vi "Laurel StandAlone TCP.vi"() -> ()   [LabVIEW 2016]
uses:
  Type Definitions/Laurel Serial Commands.ctl
  Type Definitions/Laurel Connection Type.ctl
panel:
  in  "stop":bool
  out "Single Item":dbl
  out "Gallons (Item 2)":dbl
  out "Flow Rate (Item 1)":dbl format="%.2f"
  in  "All Items Byte Count (Flow Rate)":i32=17
  in  "byte count (Individual)":i32=8
  in  "Laurel Serial Commands":T1
  out "read buffer":string
  out "Error Out 2":errorcluster
  in  "Error In 2":errorcluster
  in  "Hot Laurel Only":string="10.2.0.23"
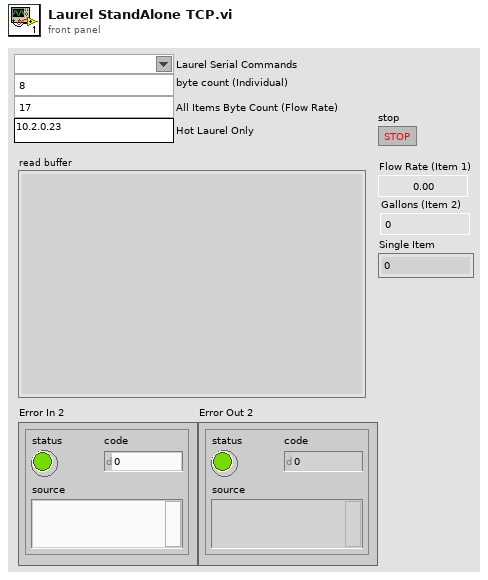
[diagram p1: front panel]
types:
  T1 = typedef "Laurel Serial Commands.ctl" = string
  T2 = typedef "Laurel Connection Type.ctl" = enum16{"Serial", "TCP"}
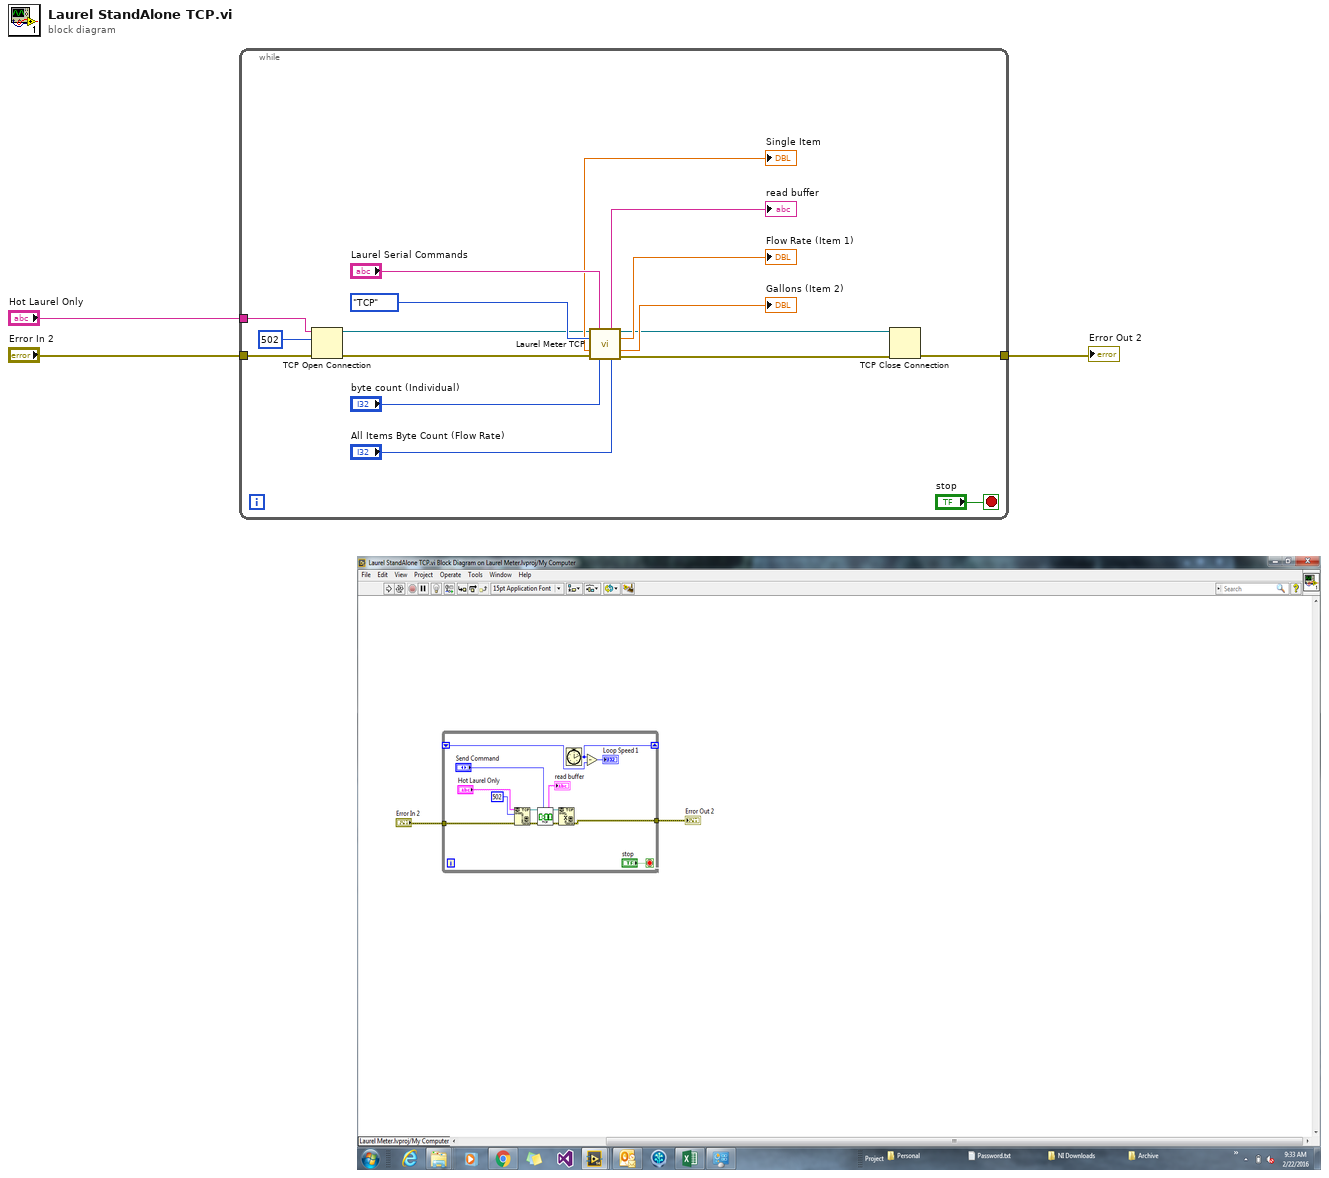
[diagram p0: block diagram]
diagram:
  n1 = while {
    tunnel: "Hot Laurel Only" -> [w9]
    tunnel: "Error In 2" -> [w8]
    tunnel: [w4] -> w1
    stop <- "stop" stop-if-true
    n2 = TCP Open Connection(address=w9, remote port or service name=u16 502, error in (no error)=w8) -> (connection ID=w7:refnum<k5>, error out=w10:errorcluster)  [unwired: 2 in]
    n3 = call "Laurel Meter TCP.vi"("TCP Network Connection in"=w7, "Laurel Serial Commands"="Laurel Serial Commands", "Connection Type"=Laurel_Connection_Type."TCP", "error in (no error)"=w10, "byte count (Individual)"="byte count (Individual)", "All Items Byte Count (Flow Rate)"="All Items Byte Count (Flow Rate)") -> ("read buffer"=→"read buffer":string, "TCP Network Connection out"=w5:refnum<k5>, "Flow Rate (Item 1)"=→"Flow Rate (Item 1)":dbl, "Single Item"=→"Single Item":dbl, "Gallons (Item 2)"=→"Gallons (Item 2)":dbl, "error out"=w6:errorcluster)  [unwired: 3 in, 1 out]
    n4 = TCP Close Connection(connection ID=w5, error in (no error)=w6) -> (error out=w4:errorcluster)  [unwired: 1 in, 1 out]
  }
  "Error Out 2" <- w1
